vi "MDrive_Init_Com.vi"(0 "VISA resource name":refnum<visa-resource-name>, 2 "baud rate":u32) -> (6 "VISA resource name out":refnum<visa-resource-name>, 8 "error out":errorcluster)   [LabVIEW 2011]
uses:
  <vilib>/Instr/_visa.llb/VISA Set IO Buffer Mask.ctl
  <vilib>/Instr/_visa.llb/VISA Configure Serial Port (Instr).vi
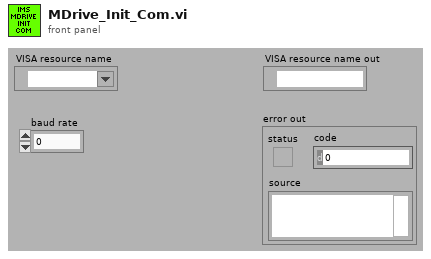
[diagram p1: front panel]
types:
  T1 = typedef "VISA Set IO Buffer Mask.ctl" = u16
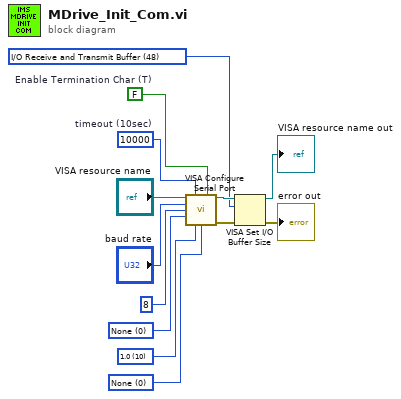
[diagram p0: block diagram]
diagram:
  w1 = u16 10 items=["1.0"=10, "1.5"=15, "2.0"=20] ("stop bits (10: 1 bit)")
  w3 = u16 0 items=["None", "Odd", "Even", "Mark", "Space"] ("parity")
  w2 = u16 0 items=["None"=0, "XON/XOFF"=1, "RTS/CTS"=2, "DTR/DSR"=4] ("flow control")
  w5 = T1 48 items=["I/O Receive Buffer"=16, "I/O Transmit Buffer"=32, "I/O Receive and Transmit Buffer"=48] ("Mask")
  w9 = FALSE  # Enable Termination Char (T)
  w6 = u32 10000  # timeout (10sec)
  n1 = call-poly "VISA Configure Serial Port"("VISA resource name"="VISA resource name", "timeout (10sec)"=w6, "Enable Termination\nChar (T)"=w9, "baud rate (9600)"="baud rate", "data bits (8)"=u16 8 ("data bits"), "parity (0:none)"=w3, "stop bits (10: 1 bit)"=w1, "flow control (0:none)"=w2) -> ("VISA resource name out"=w10:refnum<visa-resource-name>, "error out"=w11:errorcluster)  [unwired: 1 in, 5 out]
  n2 = VISA Set I/O Buffer Size(VISA resource name=w10, mask (16)=w5, error in (no error)=w11) -> (VISA resource name out=→"VISA resource name out":refnum<visa-resource-name>, error out=→"error out":errorcluster)  [unwired: 1 in]
